vi "LWXPS_DebugCorrectorTimeUsageGet.vi"(0 "XPS Reference IN":refnum<k24>, 5 "LabVIEW error IN":errorcluster) -> (7 "LabVIEW error OUT":errorcluster, 8 "XPS Reference OUT":refnum<k24>, 9 "XPS Error String":string, 10 "Returned error code":i32, 11 "ISR Init Param 2 Duration":dbl, 12 "ISR Init Param 0 Duration":dbl, 13 "ISR Gathering Duration":dbl, 14 "ISR Init Param 1 Duration":dbl, 15 "ISR Timer Duration":dbl, 16 "ISR GPIO Duration":dbl, 17 "ISR Groups Duration":dbl, 18 "ISR Event Duration":dbl, 19 "ISR General Inhib Duration":dbl)   [LabVIEW 2014]
uses:
  D:/XPSQ8_LabView_Library/Development/Source/Dll/Newport.XPS.CommandInterface.dll
  Dll/Newport.XPS.CommandInterface.dll
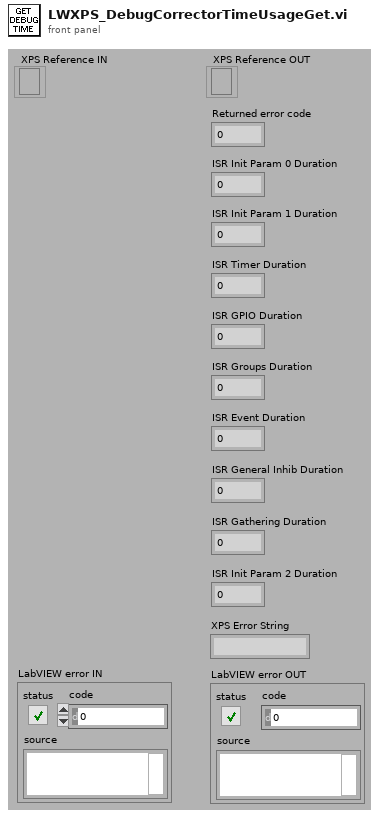
[diagram p1: front panel]
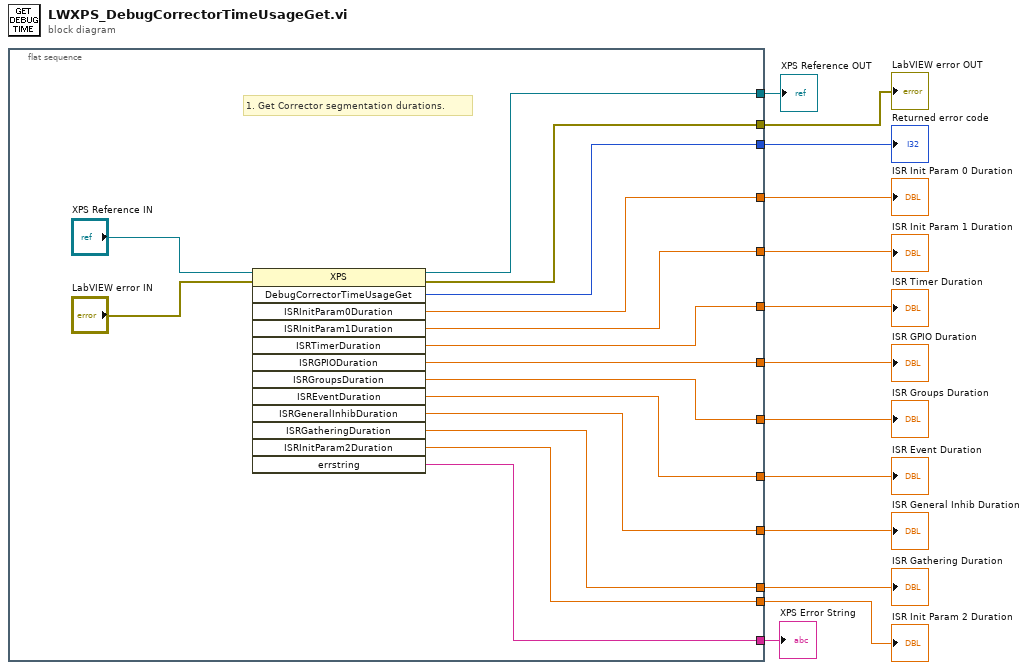
[diagram p0: block diagram]
diagram:
  n1 = flat-sequence {
    tunnel: [w26] -> w13
    tunnel: [w24] -> w12
    tunnel: [w27] -> w11
    tunnel: [w19] -> w2
    tunnel: [w22] -> w3
    tunnel: [w23] -> w6
    tunnel: [w21] -> w4
    tunnel: [w20] -> w5
    tunnel: [w18] -> w7
    tunnel: [w17] -> w8
    tunnel: [w16] -> w9
    tunnel: [w15] -> w10
    tunnel: [w14] -> w1
    frame #0 {
      # "1. Get Corrector segmentation durations."
      n2 = invoke class="XPS" method="DebugCorrectorTimeUsageGet"(reference="XPS Reference IN", error in="LabVIEW error IN") -> (reference out=w26:refnum<k24>, error out=w24:errorcluster, "DebugCorrectorTimeUsageGet"=w27:i32, "ISRInitParam0Duration"=w14:dbl, "ISRInitParam1Duration"=w19:dbl, "ISRTimerDuration"=w22:dbl, "ISRGPIODuration"=w21:dbl, "ISRGroupsDuration"=w20:dbl, "ISREventDuration"=w23:dbl, "ISRGeneralInhibDuration"=w18:dbl, "ISRGatheringDuration"=w17:dbl, "ISRInitParam2Duration"=w16:dbl, "errstring"=w15:string)  [unwired: 11 in]
    }
  }
  "XPS Error String" <- w10
  "XPS Reference OUT" <- w13
  "LabVIEW error OUT" <- w12
  "Returned error code" <- w11
  "ISR Init Param 1 Duration" <- w2
  "ISR Timer Duration" <- w3
  "ISR GPIO Duration" <- w4
  "ISR Groups Duration" <- w5
  "ISR Event Duration" <- w6
  "ISR General Inhib Duration" <- w7
  "ISR Gathering Duration" <- w8
  "ISR Init Param 2 Duration" <- w9
  "ISR Init Param 0 Duration" <- w1
